vi "Write.vi"(8 "error in (no error)":errorcluster, 9 "Timeout S (0)":dbl, 10 "Data":string, 11 "DeployResource in":refnum<class "Resource.lvclass">) -> (0 "error out":errorcluster, 2 "Bytes Written":i32, 3 "DeployResource out":refnum<class "Resource.lvclass">)   [LabVIEW 2020, in "PicoG-Core.lvlib" / "Resource.lvclass"]
uses:
  Resource.lvclass
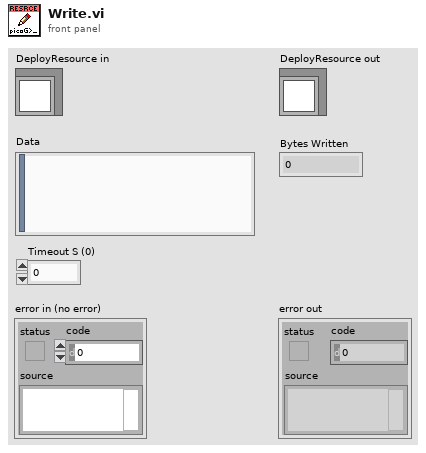
[diagram p1: front panel]
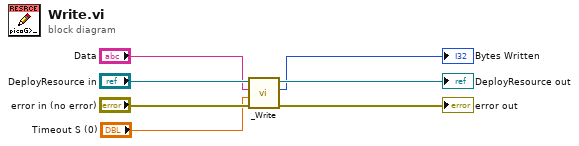
[diagram p0: block diagram]
diagram:
  n1 = call-dynamic "_Write.vi"("error in (no error)"="error in (no error)", "Timeout S (0)"="Timeout S (0)", "Data"="Data", "DeployResource in"="DeployResource in") -> ("error out"=→"error out":errorcluster, "Bytes Written"=→"Bytes Written":i32, "DeployResource out"=→"DeployResource out":refnum<class "Resource.lvclass">)  [unwired: 5 in]
